vi "ADAM_setup_ch_names.vi"() -> (0 "Ch Names":string[](array[string]))   [LabVIEW 2010]
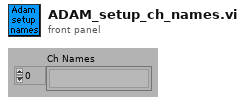
[diagram p1: front panel]
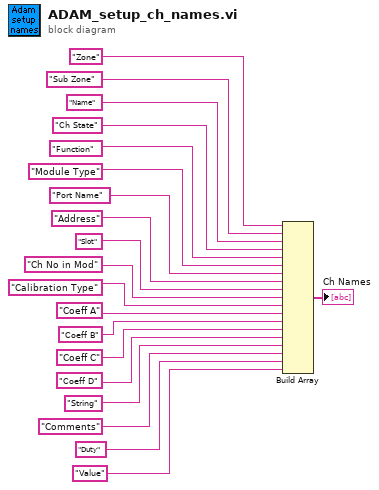
[diagram p0: block diagram]
diagram:
  n1 = Build Array("Zone" ("Label for characters"), "Sub Zone" ("Label for characters"), "Name" ("Label for characters"), "Ch State" ("Label for characters"), "Function" ("Label for characters"), "Module Type" ("Label for characters"), "Port Name", "Address" ("Label for characters"), "Slot" ("Label for characters"), "Ch No in Mod" ("Label for characters"), "Calibration Type" ("Label for characters"), "Coeff A" ("Label for characters"), "Coeff B" ("Label for characters"), "Coeff C" ("Label for characters"), "Coeff D" ("Label for characters"), "String" ("Label for characters"), "Comments" ("Label for characters"), "Duty", "Value") -> (→"Ch Names":string[])
